vi "Spectrometer Data.vi"() -> (0 "Spectrometer Data":T1={"Configuration"={"Laser Settings"={"Laser Wavelength"=enum."784 nm", "Neutral Density Filter"=enum."50%"}, "Spectrometer Settings"={"Confocal Hole Size (µm)"=150.0, "Grating"=2, "Detector"=enum."InGaAs Array"}, "Acquisition Settings"={"Acquisition Mode"=enum."Multi-Window", "Spectal Position (nm)"=632.0, "From (nm)"=735.0, "To (nm)"=3.0, "Integration Time (s)"=3.0, "Number of Accumulations"=3, "AutoScanning"=FALSE, "Spike Removal"=FALSE}, "Path"=path "C:/07 - Prizes and Awards/Marie Curie Prize/Reply Editors Final NCOMMS(10).docx"}, "Refnums"={"Instrument Status"=refnum, "Optical Spectrum Plot"={"Plot List"=refnum, "Optical Spectrum vs Energy"=refnum, "Optical Spectrum vs Wavelength"=refnum, "Optical Spectrum vs Raman Shift"=refnum, "Detector Temperature"=refnum}, "Laser"=refnum, "Filter"=refnum, "Laser ON?"=refnum, "Hole"=refnum, "Grating"=refnum, "Detector"=refnum, "Acquisition Mode"=refnum, "Spectal Position"=refnum, "From"=refnum, "To"=refnum, "Integration Time"=refnum, "Accumulations"=refnum, "AutoScanning"=refnum, "Spike Removal"=refnum, "Acquisition Mode Panel"=refnum}, "Initialization"={"Connect"=FALSE, "Update Refnums"=FALSE, "Get Configuration"=FALSE}} {"Configuration"."Spectrometer Settings"."Grating" items=["1800 l/mm", "150 l/mm"]})   [LabVIEW 2014]
uses:
  Spectrometer Data.ctl
  Spectrometer Config.ctl
  Laser Settings.ctl
  Laser.ctl
  Filter.ctl
  Grating Detector Settings.ctl
  Grating.ctl
  Detector.ctl
  Acquisition Settings.ctl
  Spectrometer Refnum.ctl
  Measurements/Plot Data/Optical Spectrum Plot Refnum.ctl
  Spectrometer Initialization.ctl
panel:
  # "LICENSED MATERIALS – PROPERTY OF IBM\nCopyright IBM Corp. 2016,\nALL RIGHTS RESERVED"
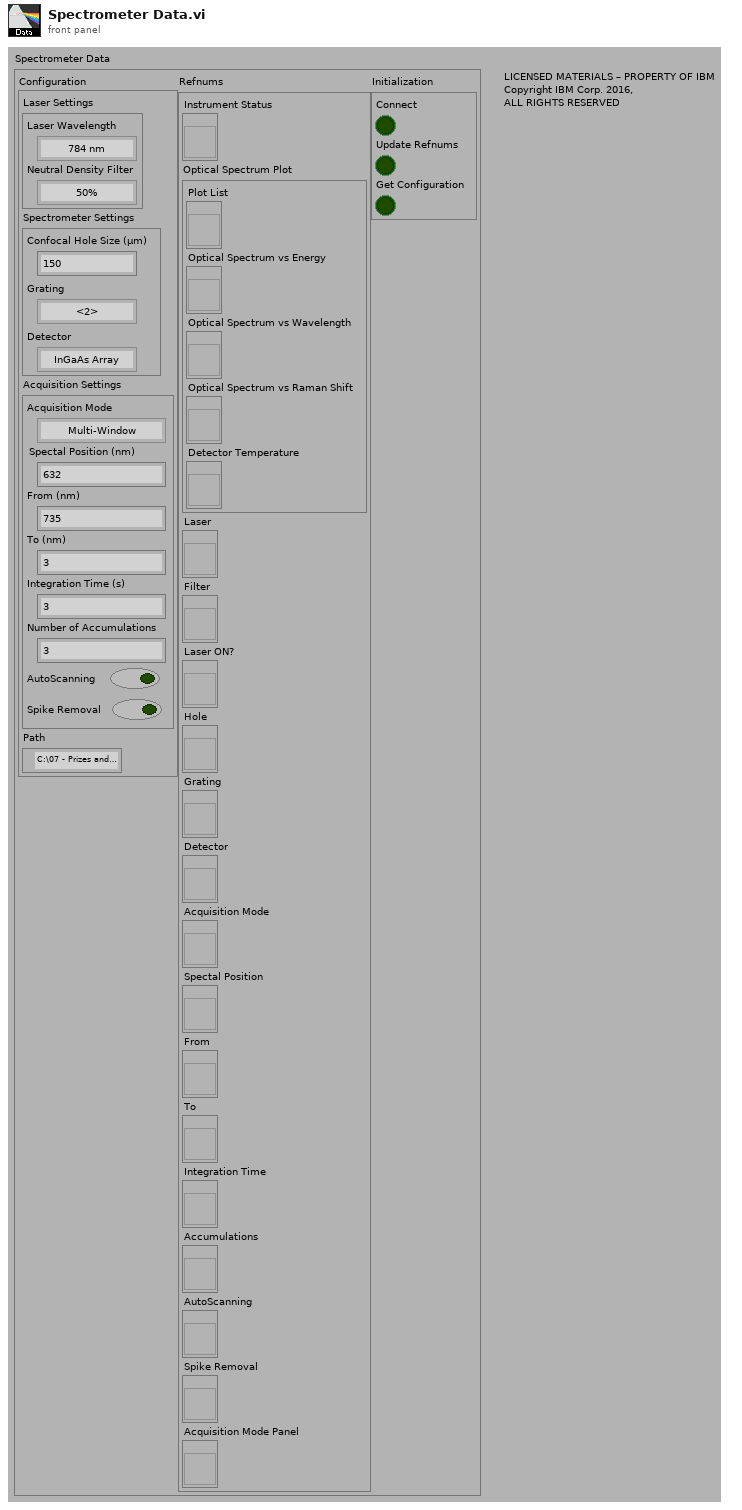
[diagram p1: front panel]
types:
  T1 = typedef "Spectrometer Data.ctl" = cluster{"Configuration":T2, "Refnums":T10, "Initialization":T12}
  T2 = typedef "Spectrometer Config.ctl" = cluster{"Laser Settings":T3, "Spectrometer Settings":T6, "Acquisition Settings":T9, "Path":path}
  T3 = typedef "Laser Settings.ctl" = cluster{"Laser Wavelength":T4, "Neutral Density Filter":T5}
  T4 = typedef "Laser.ctl" = enum16{"633 nm", "784 nm", "532 nm", "365 nm"}
  T5 = typedef "Filter.ctl" = enum16{"100%", "50%", "25%", "10%", "1%", "0.1%", "0.01%"}
  T6 = typedef "Grating Detector Settings.ctl" = cluster{"Confocal Hole Size (µm)":dbl, "Grating":T7, "Detector":T8}
  T7 = typedef "Grating.ctl" = u16
  T8 = typedef "Detector.ctl" = enum16{"InGaAs Array", "Silicon CCD"}
  T9 = typedef "Acquisition Settings.ctl" = cluster{"Acquisition Mode":enum16{"Single Window", "Multi-Window"}, "Spectal Position (nm)":dbl, "From (nm)":dbl, "To (nm)":dbl, "Integration Time (s)":dbl, "Number of Accumulations":i32, "AutoScanning":bool, "Spike Removal":bool}
  T10 = typedef "Spectrometer Refnum.ctl" = cluster{"Instrument Status":refnum<vi>, "Optical Spectrum Plot":T11, "Laser":refnum<vi>, "Filter":refnum<vi>, "Laser ON?":refnum<vi>, "Hole":refnum<vi>, "Grating":refnum<vi>, "Detector":refnum<vi>, "Acquisition Mode":refnum<vi>, "Spectal Position":refnum<vi>, "From":refnum<vi>, "To":refnum<vi>, "Integration Time":refnum<vi>, "Accumulations":refnum<vi>, "AutoScanning":refnum<vi>, "Spike Removal":refnum<vi>, "Acquisition Mode Panel":refnum<vi>}
  T11 = typedef "Optical Spectrum Plot Refnum.ctl" = cluster{"Plot List":refnum<vi>, "Optical Spectrum vs Energy":refnum<vi>, "Optical Spectrum vs Wavelength":refnum<vi>, "Optical Spectrum vs Raman Shift":refnum<vi>, "Detector Temperature":refnum<vi>}
  T12 = typedef "Spectrometer Initialization.ctl" = cluster{"Connect":bool, "Update Refnums":bool, "Get Configuration":bool}
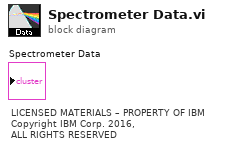
[diagram p0: block diagram]
diagram:
  # "LICENSED MATERIALS – PROPERTY OF IBM\nCopyright IBM Corp. 2016,\nALL RIGHTS RESERVED"
